vi "AVS_PollScan.vi"(9 "a_hDevice":i32) -> (3 "Output Value":i32)   [LabVIEW 2016]
uses:
  libavs.so
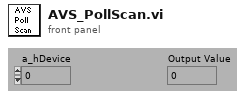
[diagram p1: front panel]
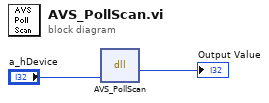
[diagram p0: block diagram]
diagram:
  n1 = dll-call lib="home/harini/tcs/ts_sedspectrometer/ss_sedspectrometer/VIs/libavs.so" fn="AVS_PollScan"("a_hDevice"="a_hDevice") -> ("return type"=→"Output Value":i32)  [unwired: 4 in, 2 out]
